vi "ConfigACBandwidth.vi"(8 "error in (no error)":errorcluster, 11 "HP3458aDMM in":refnum<class "HP3458aDMM.lvclass">) -> (0 "error out":errorcluster, 3 "HP3458aDMM out":refnum<class "HP3458aDMM.lvclass">)   [LabVIEW 2014, in "SamplerPlugins.lvlib" / "HP3458aDMM.lvclass"]
uses:
  HP3458aDMM.lvclass
  <vilib>/ErrorRing/Error Ring.xnode
  <vilib>/Utility/error.llb/Error Cluster From Error Code.vi
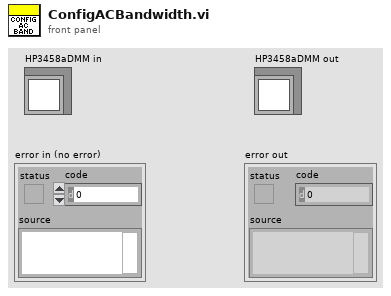
[diagram p1: front panel]
types:
  T1 = typedef "NISTSamplerPlugins.lvlib/NISTSamplerPluginsBase.lvclass/ConfigACBandwidthParams.ctl" = cluster{"dMinFreq":dbl, "dMaxFreq":dbl}
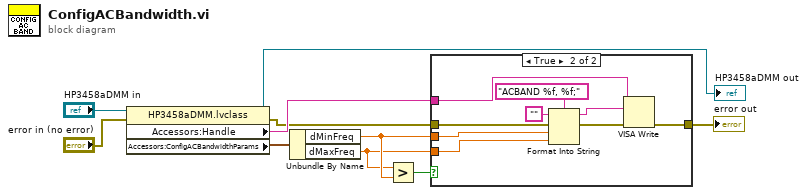
[diagram p0: block diagram]
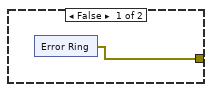
[diagram p2: hidden frame]
diagram:
  n1 = property class="HP3458aDMM.lvclass"(reference="HP3458aDMM in", error in="error in (no error)") -> (reference out=→"HP3458aDMM out":refnum<class "HP3458aDMM.lvclass">, error out=w5:errorcluster, "Accessors:Handle"=w6:string, "Accessors:ConfigACBandwidthParams"=w7:T1)
  n2 = Unbundle By Name(w7) -> ("dMinFreq"=w3:dbl, "dMaxFreq"=w2:dbl)
  n3 = Greater?(x=w2, y=w3) -> (0:w1:bool)
  n4 = case shown="True" w1 {
    tunnel: w6 -> [_ w25]
    tunnel: w5 -> [_ w24]
    tunnel: [w11 w23] -> w4
    tunnel: w3 -> [_ w18]
    tunnel: w2 -> [_ w17]
    frame False {
      n5 = xnode "Error Ring"() -> ("error out"=w11:errorcluster)
    }
    frame True {
      n6 = Format Into String(format string="ACBAND %f, %f;", initial string="", error in=w24, w18, w17) -> (resulting string=w19:string, error out=w22:errorcluster)
      n7 = VISA Write(VISA resource name=w25, write buffer=w19, error in (no error)=w22) -> (error out=w23:errorcluster)  [unwired: 2 out]
    }
  }
  "error out" <- w4
